vi "Strip Whitespace.vi"(8 "Error In":errorcluster, 11 "Text":string) -> (0 "Error Out":errorcluster, 3 "Stripped Text":string)   [LabVIEW 2015, in "Logger.lvlib"]
uses:
  Logger.lvlib
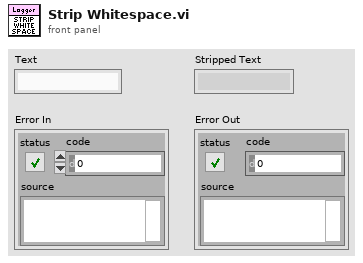
[diagram p1: front panel]
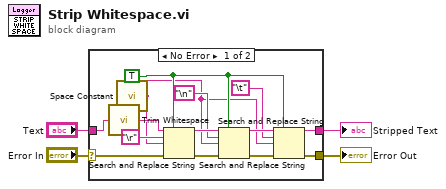
[diagram p0: block diagram]
diagram:
  n1 = case shown="No Error" "Error In" {
    selector: "Error In" -> [w12 w20]
    tunnel: [w10 w20] -> w4
    tunnel: "Text" -> [w13 w19]
    tunnel: [w8 w19] -> w1
    frame No Error {
      w7 = TRUE ("replace all? (F)")
      n2 = call <vilib>:"Trim Whitespace.vi"("string"=w13) -> ("trimmed string"=w18:string)  [unwired: 1 in]
      n3 = call <vilib>:"Space Constant.vi"() -> ("String"=w5:string)
      n4 = Search and Replace String(replace all?=w7, input string=w18, search string="\r", replace string=w5, error in=w12) -> (result string=w16:string, error out=w14:errorcluster)  [unwired: 3 in, 2 out]
      n5 = Search and Replace String(replace all?=w7, input string=w16, search string="\n", replace string=w5, error in=w14) -> (result string=w9:string, error out=w11:errorcluster)  [unwired: 3 in, 2 out]
      n6 = Search and Replace String(replace all?=w7, input string=w9, search string="\t", replace string=w5, error in=w11) -> (result string=w8:string, error out=w10:errorcluster)  [unwired: 3 in, 2 out]
    }
    frame Error {
    }
  }
  "Error Out" <- w4
  "Stripped Text" <- w1
